vi "InvokeEventByIdAndCategory.vi"(0 "ID":string, 1 "Category":string, 5 "eventName":string, 7 "Data":variant, 9 "Invoke? (t)":bool=TRUE, 11 "error in (no error)":errorcluster) -> (15 "error out":errorcluster)   [LabVIEW 2017]
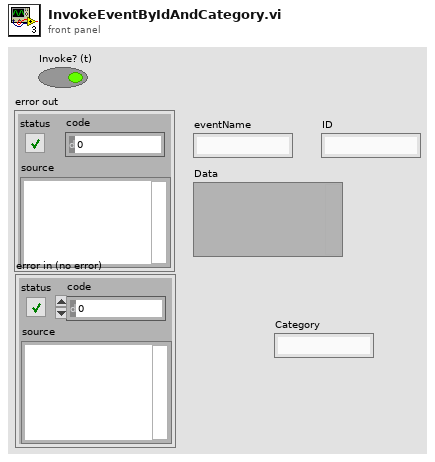
[diagram p1: front panel]
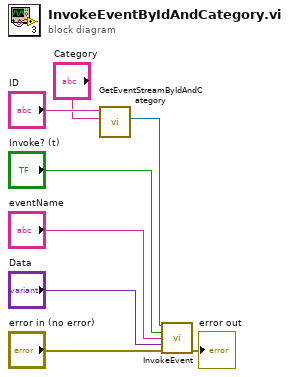
[diagram p0: block diagram]
diagram:
  n1 = call "GetEventStreamByIdAndCategory.vi"("Category"="Category", "ID"="ID") -> ("Event Stream Out"=w2:refnum<user-event>)  [unwired: 7 in, 2 out]
  n2 = call "InvokeEvent.vi"("Event Stream In"=w2, "Invoke?"="Invoke? (t)", "name"="eventName", "Data"="Data", "error in (no error)"="error in (no error)") -> ("error out"=→"error out":errorcluster)  [unwired: 9 in, 1 out]
